vi "GetLastTrend.vi"(7 "LabVIEW Web Service Request":refnum<class "Web Request.lvclass">, 11 "MetricID":string) -> (3 "LastTrend":cluster{"String":string, "Value":dbl})   [LabVIEW 2017]
uses:
  <vilib>/wsapi/Web Request.lvclass
  typedefs/Q_Message.ctl
panel:
  # "Use the Web Service Request input terminal to call the VIs on the Web Services palette. Do not remove it from the connector pane unless you don't need access to the palette."
  # "Each additional control wired to the connector pane will be available as an input in the URL. To include an indicator in terminal-mode output (the default setting), it must also be wired to the connector pane."
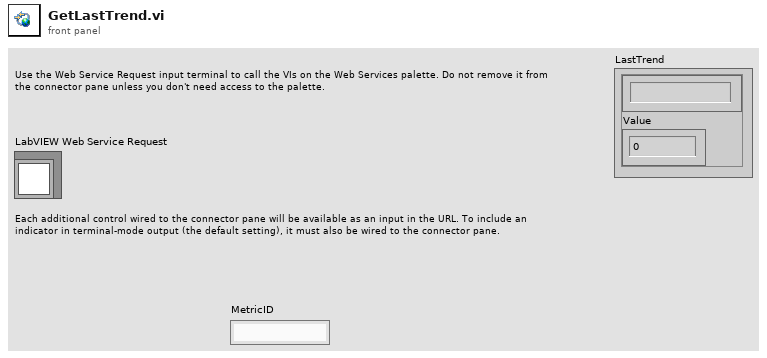
[diagram p1: front panel]
types:
  T1 = typedef "Q_Message.ctl" = cluster{"Command":string, "Parameters":variant}
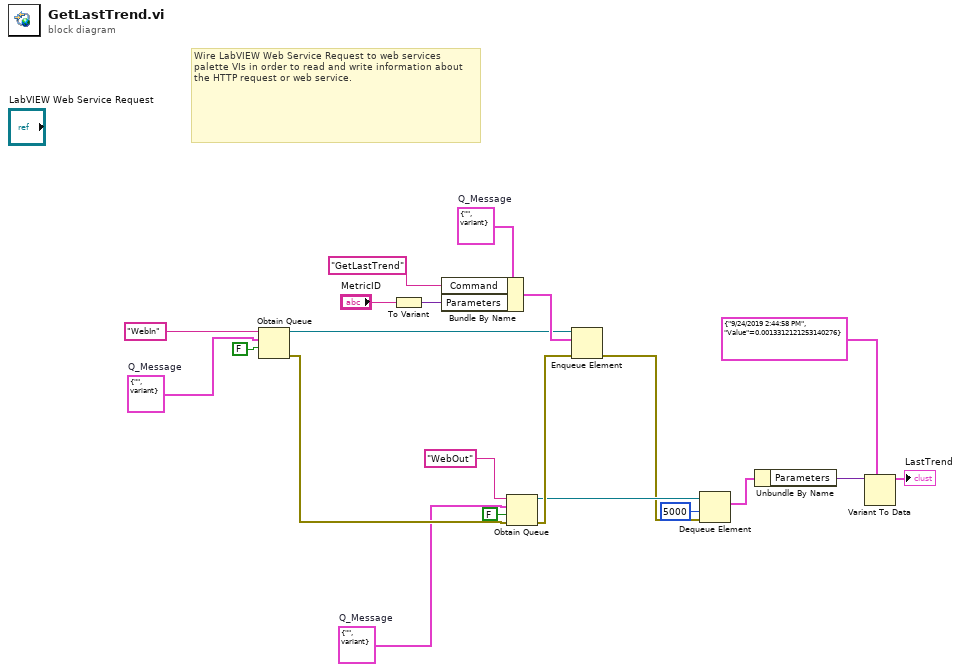
[diagram p0: block diagram]
diagram:
  w5 = T1 {"Command"="", "Parameters"=variant}  # Q_Message
  w6 = T1 {"Command"="", "Parameters"=variant}  # Q_Message
  w7 = T1 {"Command"="", "Parameters"=variant}  # Q_Message
  # "Wire LabVIEW Web Service Request to web services palette VIs in order to read and write information about the HTTP request or web service."
  n1 = Obtain Queue(name (unnamed)="WebIn", element data type=w7, create if not found? (T)=FALSE) -> (queue out=w16:refnum<queue>, error out=w13:errorcluster)  [unwired: 2 in, 1 out]
  n2 = To Variant(anything="MetricID") -> (Variant=w19:variant)
  n3 = Bundle By Name(cluster=w6, "Command"="GetLastTrend", "Parameters"=w19) -> (w18:T1)
  n4 = Obtain Queue(name (unnamed)="WebOut", element data type=w5, create if not found? (T)=FALSE, error in (no error)=w13) -> (queue out=w10:refnum<queue>, error out=w11:errorcluster)  [unwired: 1 in, 1 out]
  n5 = Enqueue Element(queue=w16, element=w18, error in (no error)=w11) -> (error out=w9:errorcluster)  [unwired: 1 in, 2 out]
  n6 = Dequeue Element(queue=w10, timeout in ms (-1)=5000, error in (no error)=w9) -> (element=w4:T1)  [unwired: 3 out]
  n7 = Unbundle By Name(w4) -> ("Parameters"=w3:variant)
  n8 = Variant To Data(type=cluster{string, "Value":dbl} {"9/24/2019 2:44:58 PM", "Value"=0.0013312121253140276} ("LastTrendPoint"), Variant=w3) -> (data=→"LastTrend":cluster{string, "Value":dbl})  [unwired: 1 in, 1 out]
